vi "action.vi"(0 "MoAgSy_Visitor_travel in":refnum<class "MoAgSy_Visitor_travel.lvclass">, 2 "HGF_Visitable":refnum<class "HGF_Visitable.lvclass">, 5 "error in (no error)":errorcluster) -> (14 "MoAgSy_Visitor_travel out":refnum<class "MoAgSy_Visitor_travel.lvclass">, 16 "dup HGF_Visitable":refnum<class "HGF_Visitable.lvclass">, 19 "error out":errorcluster)   [LabVIEW 2009, in "MoAgSy.lvlib" / "MoAgSy_Visitor_travel.lvclass"]
doc: "This is a dynamic dispatch VI that is called from Visitor.visit(). It will call member VIs of Visitable to perform the requested action which means: calling public methods of Visitable child class.\n\n<B>Hint:</B> This method is abstract and need to be implemented by child classes."
uses:
  MoAgSy_Visitor_travel.lvclass
  HGF_BaseClasses/HGF_Visitable/HGF_Visitable.lvclass
  MoAgSy_AgentBase/MoAgSy_AgentBase.lvclass
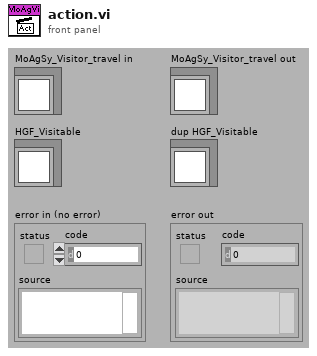
[diagram p1: front panel]
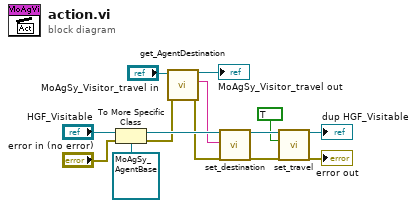
[diagram p0: block diagram]
diagram:
  n1 = To More Specific Class(target class=refnum<class "MoAgSy_AgentBase.lvclass"> refnum ("HGF_AgentBaseClasses.lvlib:HGF_Agent.lvclass"), reference="HGF_Visitable", error in="error in (no error)") -> (specific class reference=w12:refnum<class "MoAgSy_AgentBase.lvclass">, error out=w7:errorcluster)
  n2 = call "get_AgentDestination.vi"("error in (no error)"=w7, "MoAgSy_Visitor_travel.lvclass in"="MoAgSy_Visitor_travel in") -> ("error out"=w6:errorcluster, "destination"=w9:string, "MoAgSy_Visitor_travel.lvclass out"=→"MoAgSy_Visitor_travel out":refnum<class "MoAgSy_Visitor_travel.lvclass">)  [unwired: 7 out]
  n3 = call "set_destination.vi"("HGF_Agent in"=w12, "destination"=w9, "error in (no error)"=w6) -> ("HGF_Agent out"=w5:refnum<class "MoAgSy_AgentBase.lvclass">, "error out"=w2:errorcluster)  [unwired: 15 out]
  n4 = call "set_travel.vi"("HGF_Agent in"=w5, "travel?"=TRUE, "error in (no error)"=w2) -> ("HGF_Agent out"=→"dup HGF_Visitable":refnum<class "MoAgSy_AgentBase.lvclass">, "error out"=→"error out":errorcluster)  [unwired: 15 out]
